vi "SubVelocity.vi"(4 "Vessel Diameter":dbl[](array[numeric]), 5 "AVI Path":path, 6 "error in (no error)":errorcluster, 7 "Calibration factor (1 pix = ? um)":dbl=1.45, 8 "Y":dbl[](array[numeric]), 9 "X":dbl[](array[numeric])) -> (0 "error out":errorcluster, 3 "Velocity":dbl[](array[numeric]))   [LabVIEW 2017]
uses:
  <vilib>/vision/NI_Vision_Development_Module.lvlib
panel:
  in  "Search Window Width":dbl=65.0
  in  "Template Window Width":dbl=22.0
  in  "Search Window Seperation Height":dbl=10.0
  out "Particle Velocity - Unfiltered":dbl[](graph)
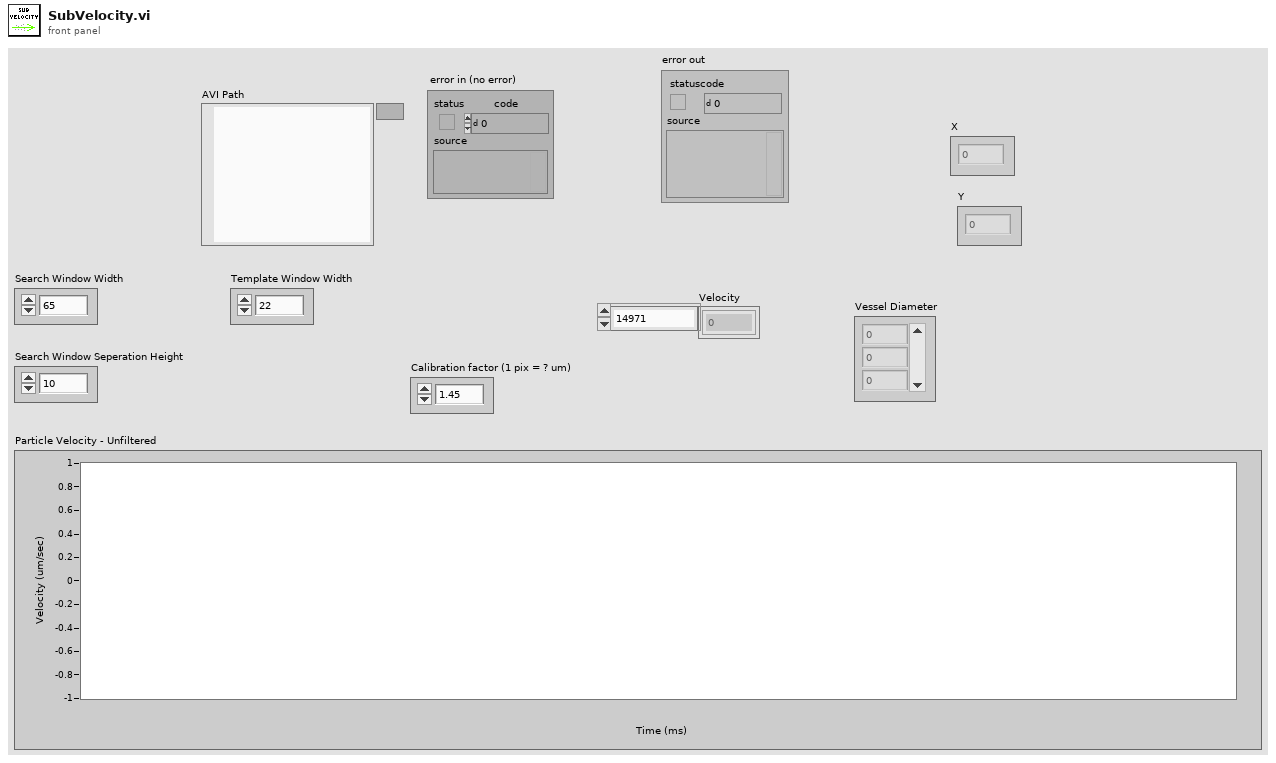
[diagram p1: front panel]
types:
  T1 = typedef "IMAQ AVI2 Refnum.ctl" = refnum<k20>
  T2 = typedef "IMAQ Image.ctl" = refnum<image>
  T3 = typedef "ROI Descriptor" = cluster{"Global Rectangle":i32[], "Contours":cluster{"ID":enum32{"External", "Internal"}, "Type":u32, "Coordinates":i32[]}[]}
  T4 = cluster{"Position":cluster{"x":sgl, "y":sgl}, "Angle":sgl, "Scale":sgl, "Score":sgl, "Bounding Box":cluster{"x":sgl, "y":sgl}[]}[]
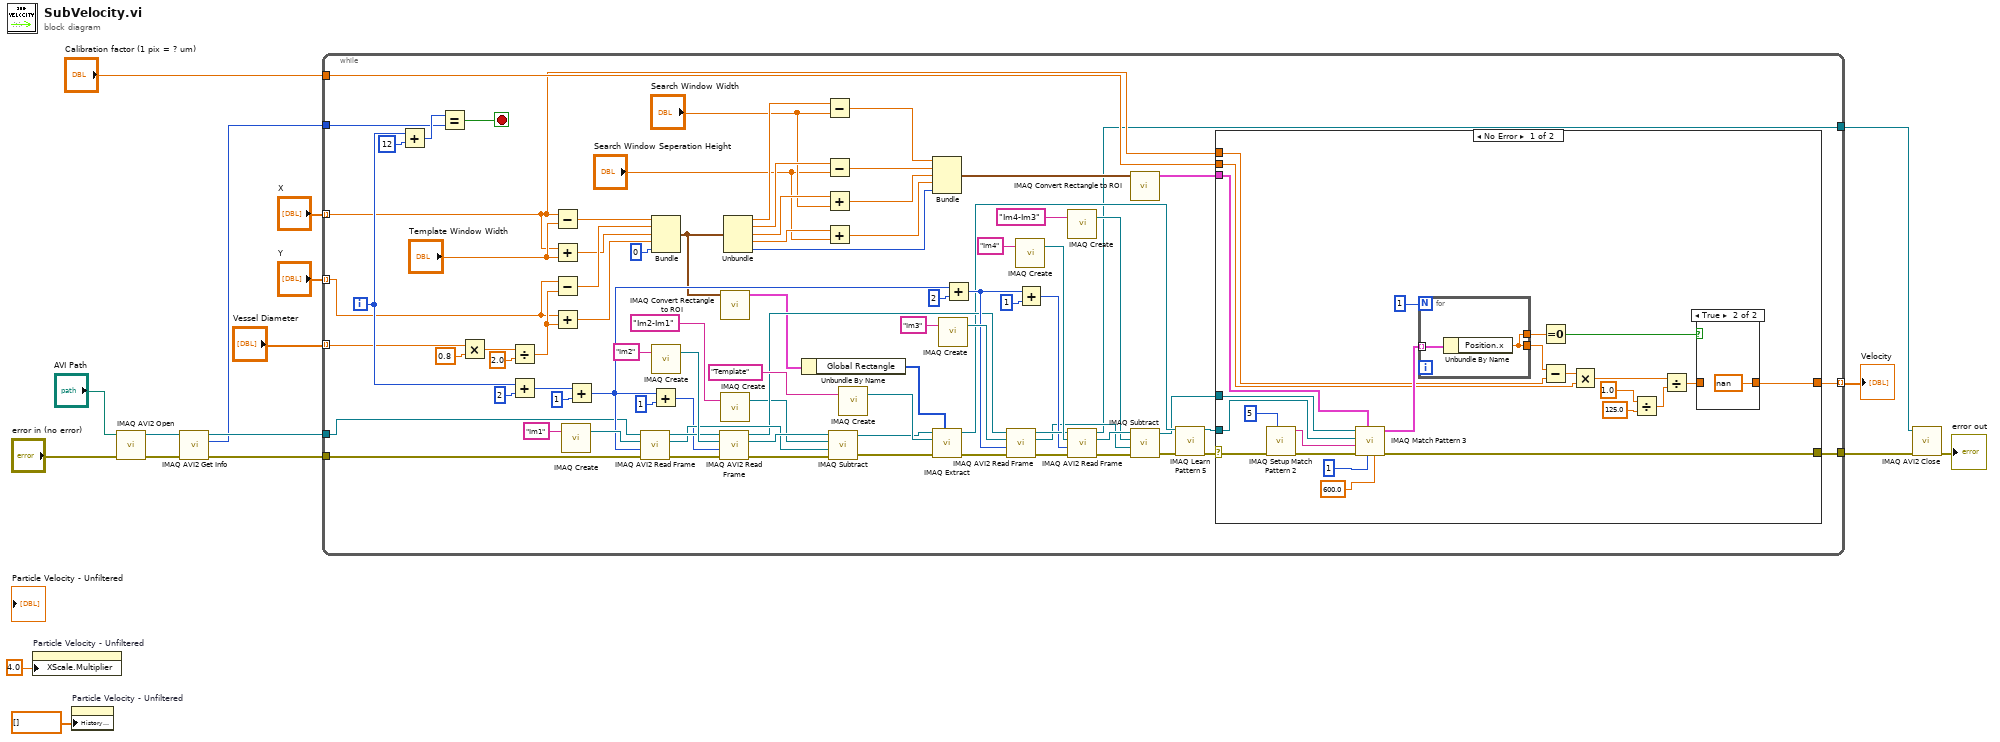
[diagram p0: block diagram]
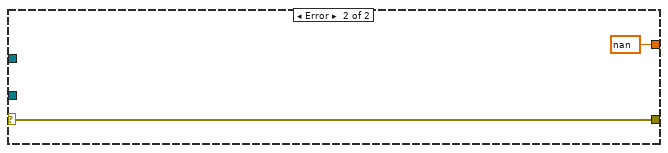
[diagram p3: hidden frame]
diagram:
  n1 = property on="Particle Velocity - Unfiltered" class="WFChart (strict)"("XScale.Multiplier"=4.0 ("X Scale.Offset and Multiplier:Multiplier")) -> ()  [unwired: 2 in, 2 out]
  n2 = property on="Particle Velocity - Unfiltered" class="WFChart (strict)"("History Data"=dbl[] []) -> ()  [unwired: 2 in, 2 out]
  n3 = call "IMAQ AVI2 Open"("error in (no error)"="error in (no error)", "AVI File Path"="AVI Path") -> ("error out"=w16:errorcluster, "AVI Refnum"=w17:T1)  [unwired: 8 in]
  n4 = call "IMAQ AVI2 Get Info"("error in (no error)"=w16, "AVI Refnum"=w17) -> ("error out"=w14:errorcluster, "Number of Frames"=w11:u32, "AVI Refnum (duplicate)"=w13:T1)  [unwired: 5 in, 2 out]
  n5 = while {
    tunnel: "Calibration factor (1 pix = ? um)" -> [w71]
    tunnel: "Vessel Diameter" -> [w31] mode=indexing
    tunnel: w14 -> [w52]
    tunnel: w13 -> [w51]
    tunnel: w11 -> [w45]
    tunnel: [w28] -> w5 mode=indexing
    tunnel: [w27] -> w3
    tunnel: "X" -> [w26] mode=indexing
    tunnel: "Y" -> [w25] mode=indexing
    tunnel: [w18] -> w2
    i -> [w34]
    stop <- w29 stop-if-true
    n6 = Add(x=w34, y=12) -> (x+y=w46:i32)
    n7 = Equal?(x=w46, y=w45) -> (x = y?=w29:bool)
    n8 = Multiply(x=w31, y=0.8) -> (x*y=w66:dbl)
    n9 = Divide(x=w66, y=2.0) -> (x/y=w70:dbl)
    n10 = Add(x=w34, y=2) -> (x+y=w32:i32)
    n11 = Subtract(x=w26, y="Template Window Width") -> (x-y=w63:dbl)
    n12 = Add(x=w26, y="Template Window Width") -> (x+y=w64:dbl)
    n13 = Subtract(x=w25, y=w70) -> (x-y=w68:dbl)
    n14 = Add(x=w25, y=w70) -> (x+y=w69:dbl)
    n15 = call "IMAQ Create"("Image Name"="Im1") -> ("New Image"=w92:T2)  [unwired: 4 in, 1 out]
    n16 = Add(x=w32, y=1) -> (x+y=w79:i32)
    n17 = call "IMAQ AVI2 Read Frame"("error in (no error)"=w52, "Frame Number"=w79, "Image"=w92, "AVI Refnum"=w51) -> ("error out"=w96:errorcluster, "Image Out"=w88:T2, "AVI Refnum (duplicate)"=w90:T1)  [unwired: 5 in]
    n18 = Add(x=w79, y=1) -> (x+y=w78:i32)
    n19 = Bundle(w63, w68, w64, w69, 0) -> (w19:cluster{dbl, dbl, dbl, dbl, i32})  [unwired: 1 in]
    n20 = call "IMAQ Create"("Image Name"="Im2") -> ("New Image"=w91:T2)  [unwired: 4 in, 1 out]
    n21 = call "IMAQ AVI2 Read Frame"("error in (no error)"=w96, "Frame Number"=w78, "Image"=w91, "AVI Refnum"=w90) -> ("error out"=w82:errorcluster, "Image Out"=w89:T2, "AVI Refnum (duplicate)"=w74:T1)  [unwired: 5 in]
    n22 = call "IMAQ Convert Rectangle to ROI"("Rectangle"=w19) -> ("ROI Descriptor"=w61:T3)  [unwired: 8 in, 1 out]
    n23 = call "IMAQ Create"("Image Name"="Im2-Im1") -> ("New Image"=w38:T2)  [unwired: 4 in, 1 out]
    n24 = Unbundle(w19) -> (w53:dbl, w50:dbl, w49:dbl, w48:dbl, w55:i32)
    n25 = Unbundle By Name(w61) -> ("Global Rectangle"=w60:i32[])
    n26 = Subtract(x=w53, y="Search Window Width") -> (x-y=w59:dbl)
    n27 = Subtract(x=w50, y="Search Window Seperation Height") -> (x-y=w57:dbl)
    n28 = Add(x=w49, y="Search Window Width") -> (x+y=w58:dbl)
    n29 = Add(x=w48, y="Search Window Seperation Height") -> (x+y=w56:dbl)
    n30 = call "IMAQ Subtract"("Image Src A"=w89, "Image Dst"=w38, "Image Src B"=w88, "error in (no error)"=w82) -> ("Image Dst Out"=w23:T2, "error out"=w22:errorcluster)  [unwired: 3 in]
    n31 = call "IMAQ Create"("Image Name"="Template") -> ("New Image"=w99:T2)  [unwired: 4 in, 1 out]
    n32 = Bundle(w59, w57, w58, w56, w55) -> (w24:cluster{dbl, dbl, dbl, dbl, i32})  [unwired: 1 in]
    n33 = call "IMAQ Extract"("Optional Rectangle"=w60, "error in (no error)"=w22, "Image Dst"=w99, "Image Src"=w23) -> ("error out"=w73:errorcluster, "Image Dst Out"=w41:T2)  [unwired: 6 in]
    n34 = call "IMAQ Create"("Image Name"="Im3") -> ("New Image"=w85:T2)  [unwired: 4 in, 1 out]
    n35 = Add(x=w79, y=2) -> (x+y=w76:i32)
    n36 = call "IMAQ AVI2 Read Frame"("error in (no error)"=w73, "Frame Number"=w76, "Image"=w85, "AVI Refnum"=w74) -> ("error out"=w95:errorcluster, "Image Out"=w39:T2, "AVI Refnum (duplicate)"=w83:T1)  [unwired: 5 in]
    n37 = call "IMAQ Create"("Image Name"="Im4") -> ("New Image"=w84:T2)  [unwired: 4 in, 1 out]
    n38 = Add(x=w76, y=1) -> (x+y=w75:i32)
    n39 = call "IMAQ Create"("Image Name"="Im4-Im3") -> ("New Image"=w36:T2)  [unwired: 4 in, 1 out]
    n40 = call "IMAQ AVI2 Read Frame"("error in (no error)"=w95, "Frame Number"=w75, "Image"=w84, "AVI Refnum"=w83) -> ("error out"=w81:errorcluster, "Image Out"=w40:T2, "AVI Refnum (duplicate)"=w18:T1)  [unwired: 5 in]
    n41 = call "IMAQ Convert Rectangle to ROI"("Rectangle"=w24) -> ("ROI Descriptor"=w54:T3)  [unwired: 8 in, 1 out]
    n42 = call "IMAQ Subtract"("Image Src A"=w40, "Image Dst"=w36, "Image Src B"=w39, "error in (no error)"=w81) -> ("Image Dst Out"=w21:T2, "error out"=w20:errorcluster)  [unwired: 3 in]
    n43 = call "IMAQ Learn Pattern 5"("Image"=w41, "error in (no error)"=w20) -> ("Template Image Out"=w72:T2, "error out"=w30:errorcluster)  [unwired: 11 in, 1 out]
    n44 = case shown="No Error" w30 {
      selector: w30 -> [w124 w130]
      tunnel: w72 -> [w122 _]
      tunnel: w71 -> [w118 _]
      tunnel: [w101 w130] -> w27
      tunnel: w54 -> [w117 _]
      tunnel: w26 -> [w111 _]
      tunnel: [w112 nan] -> w28
      tunnel: w21 -> [w102 _]
      frame No Error {
        n45 = call "IMAQ Setup Match Pattern 2"("Minimum Contrast"=5, "error in (no error)"=w124) -> ("error out"=w115:errorcluster, "Match Pattern Setup Data"=w116:string)  [unwired: 8 in]
        n46 = call "IMAQ Match Pattern 3"("Minimum Match Score"=sgl 600.0, "Number of Matches Requested"=1, "ROI Descriptor"=w117, "error in (no error)"=w115, "Match Pattern Setup Data"=w116, "Template Image"=w122, "Image"=w102) -> ("error out"=w101:errorcluster, "Matches"=w120:T4)  [unwired: 2 in, 1 out]
        n47 = for {
          N: 1 -> [_]
          tunnel: [w127] -> w110
          tunnel: w120 -> [w128] mode=indexing
          tunnel: [w127] -> w113
          n48 = Unbundle By Name(w128) -> ("Position.x"=w127:sgl)
        }
        n49 = Equal To 0?(x=w113) -> (x = 0?=w114:bool)
        n50 = Subtract(x=w110, y=w111) -> (x-y=w119:dbl)
        n51 = Multiply(x=w119, y=w118) -> (x*y=w106:dbl)
        n52 = Divide(x=1.0, y=125.0) -> (x/y=w107:dbl)
        n53 = Divide(x=w106, y=w107) -> (x/y=w105:dbl)
        n54 = case shown="True" w114 {
          tunnel: [w125 nan] -> w112
          tunnel: w105 -> [w125 _]
          frame False {
          }
          frame True {
          }
        }
      }
      frame Error {
      }
    }
  }
  "Velocity" <- w5
  n55 = call "IMAQ AVI2 Close"("error in (no error)"=w3, "AVI Refnum"=w2) -> ("error out"=→"error out":errorcluster)  [unwired: 9 in]
